vi "Actor Core.vi"(8 "error in":errorcluster, 11 "Panel Actor With Events in":refnum<class "Helper Methods.lvclass">) -> (0 "error out":errorcluster, 3 "Actor out":refnum<class "Actor.lvclass">)   [LabVIEW 2017, in "2. Basic Panel Actors.lvlib" / "Helper Methods.lvclass"]
doc: "The user interface for this panel.\n----\nCopyright: MGI 2016\nAuthor: Derek Trepanier"
uses:
  Helper Methods.lvclass
  <vilib>/ActorFramework/Stop Msg/Stop Msg.lvclass
  panel-manager/Source/MGI-Panel Manager.lvlib
  panel-manager/Source/Panel/Subpanel/Subpanel.vi
  panel-manager/Source/Panel/Subpanel/Subpanel.lvclass
  Description Panel/Description Panel.lvclass
  panel-actors/Source/Panel Actor/Panel Actor.lvclass
  D:/test/LabView_PanelManager/panel-actors/Source/Panel Actor/Panel Actor.lvclass
  D:/test/LabView_PanelManager/panel-manager/Source/Panel/Panel.lvclass
  <vilib>/ActorFramework/Actor/Actor.lvclass
panel:
  out "Initialization Time":string
  out "Latest ID":i32
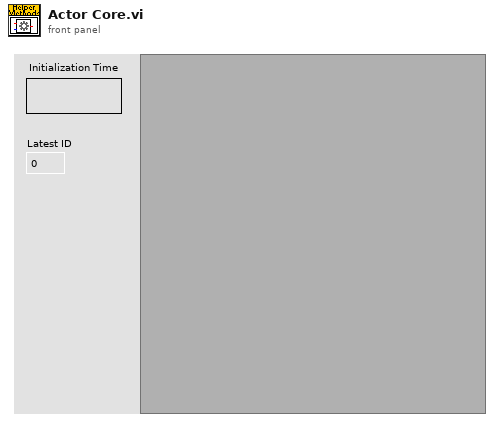
[diagram p1: front panel]
types:
  T1 = cluster{"Event Registration Refnum":refnum<event-registration>, "Pnl Actor":refnum<event-registration>}
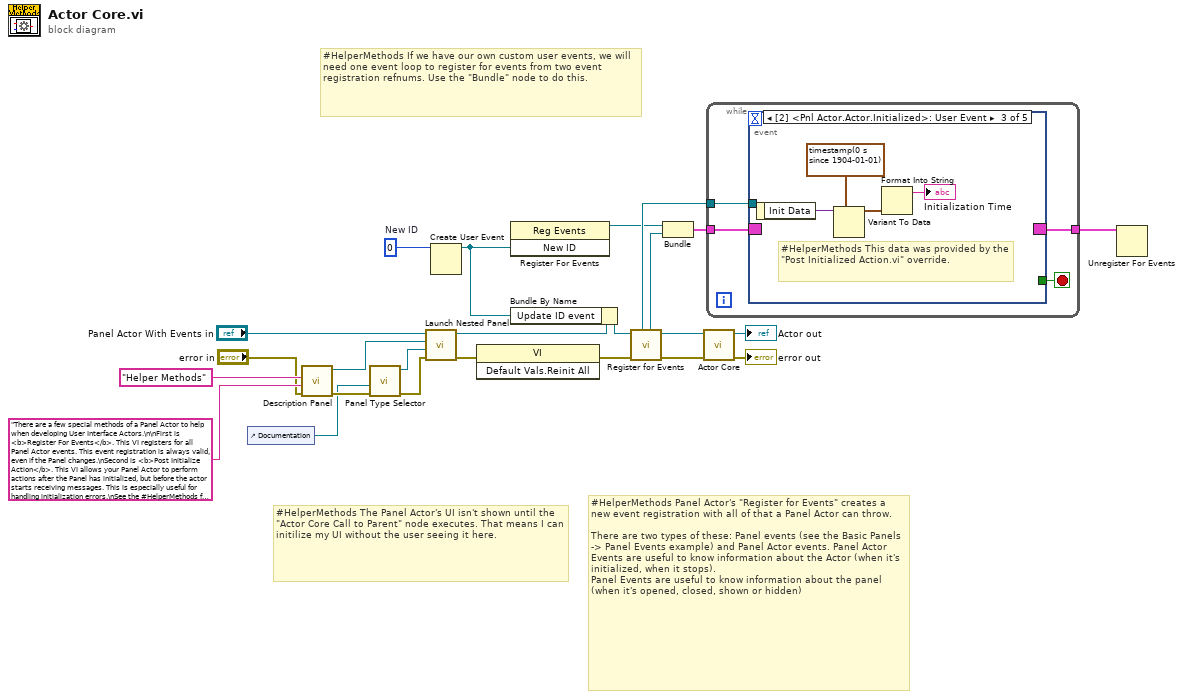
[diagram p0: block diagram]
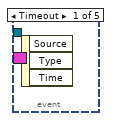
[diagram p2: hidden frame]
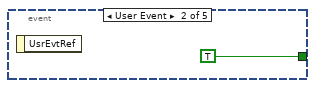
[diagram p3: hidden frame]
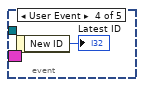
[diagram p4: hidden frame]
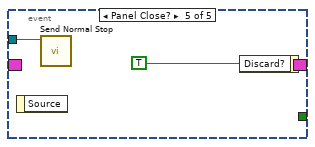
[diagram p5: hidden frame]
diagram:
  w17 = 0  # New ID
  # "#HelperMethods The Panel Actor's UI isn't shown until the \"Actor Core Call to Parent\" node executes. That means I can initilize my UI without the user seeing it here."
  # "#HelperMethods If we have our own custom user events, we will need one event loop to register for events from two event registration refnums. Use the \"Bundle\" node to do this."
  # "#HelperMethods Panel Actor's \"Register for Events\" creates a new event registration with all of that a Panel Actor can throw.\n\nThere are two types of these: Panel events (see the Basic Panels -> Panel Events example) and Panel Actor events. Panel Actor Events are useful to know information about the Actor (when it's initialized, when it stops).\nPanel Events are useful to know information about the panel (when it's opened, closed, shown or hidden)"
  n1 = control-ref of="Documentation"() -> (w1:refnum<vi>)
  n2 = call "Description Panel.vi"("error in (no error)"="error in", "Description"="There are a few special methods of a Panel Actor to help when developing User Interface Actors.\n\nFirst is <b>Register For Events</b>. This VI registers for all Panel Actor events. This event registration is always valid, even if the Panel changes.\nSecond is <b>Post Initialize Action</b>. This VI allows your Panel Actor to perform actions after the Panel has initialized, but before the actor starts receiving messages. This is especially useful for handling initialization errors.\nSee the #HelperMethods for more info.\n" ("Description Title"), "Description Title"="Helper Methods") -> ("error out"=w5:errorcluster, "Description Panel out"=w9:refnum<class "Description Panel.lvclass">)  [unwired: 7 in]
  n3 = call-poly "Panel Type Selector.vi"("Error In"=w5, "Sub Panel"=w1) -> ("Error Out"=w10:errorcluster, "Subpanel Out"=w11:refnum<class "Subpanel.lvclass">)  [unwired: 8 in]
  n4 = call "Launch Nested Panel.vi"("error in (no error)"=w10, "Panel"=w11, "Nested Panel Actor"=w9, "Panel Actor in"="Panel Actor With Events in") -> ("error out"=w2:errorcluster, "Panel Actor out"=w3:refnum<class "Helper Methods.lvclass">)  [unwired: 4 in, 2 out]
  n5 = Create User Event(user event datatype=w17) -> (user event=w13:refnum<user-event>)  [unwired: 1 in, 1 out]
  n6 = invoke class="VI" method="Default Vals.Reinit All"(error in=w2) -> (error out=w12:errorcluster)  [unwired: 2 in, 2 out]
  n7 = register-events(w13) -> (reference out=w15:refnum<event-registration>)  [unwired: 2 in, 1 out]
  n8 = Bundle By Name(cluster=w3, "Update ID event"=w13) -> (w14:refnum<class "Helper Methods.lvclass">)
  n9 = call "Register for Events.vi"("Error In"=w12, "Panel Actor in"=w14) -> ("Error Out"=w20:errorcluster, "Panel Actor out"=w21:refnum<class "Helper Methods.lvclass">, "Pnl Actor"=w19:refnum<event-registration>, "Self Enqueuer"=w18:refnum<class "Message Enqueuer.lvclass">)  [unwired: 5 in, 1 out]
  n10 = Bundle("Event Registration Refnum"=w15, "Pnl Actor"=w19) -> (w16:T1)  [unwired: 1 in]
  n11 = call-parent "Actor Core.vi"("error in"=w20, "Panel Actor in"=w21) -> ("error out"=→"error out":errorcluster, "Actor out"=→"Actor out":refnum<class "Actor.lvclass">)  [unwired: 8 in]
  n12 = while {
    tunnel: w16 -> [w28]
    tunnel: w18 -> [w27]
    tunnel: [w25] -> w22
    stop <- w26 stop-if-true
    n13 = event shown="[2] <Pnl Actor.Actor.Initialized>: User Event" {
      selector: w28 -> [_ _ _ _ _]
      dyn-events: [_ _ _ _ _] -> w25
      timeout: _ -> [_ _ _ _ _]
      tunnel: w27 -> [_ _ _ _ w36]
      tunnel: [_ TRUE _ _ _] -> w26
      event Timeout {
        n14 = event-data() -> ()  [unwired: 1 in, 3 out]
      }
      event User Event {
        n15 = event-data() -> ()  [unwired: 1 in, 1 out]
      }
      event User Event {
        # "#HelperMethods This data was provided by the \"Post Initialized Action.vi\" override."
        n16 = event-data() -> ("Init Data"=w33:variant)  [unwired: 1 in]
        n17 = Variant To Data(type=timestamp(0 s since 1904-01-01), Variant=w33) -> (data=w32:timestamp)  [unwired: 1 in, 1 out]
        n18 = Format Into String(w32) -> (resulting string=→"Initialization Time":string)  [unwired: 3 in, 1 out]
      }
      event User Event {
        n19 = event-data() -> ("New ID"=→"Latest ID":i32)  [unwired: 1 in]
      }
      event Panel Close? {
        n20 = event-data() -> ()  [unwired: 1 in, 1 out]
        n21 = call <vilib>:"Send Normal Stop.vi"("Message Enqueuer"=w36) -> ()  [unwired: 10 in, 1 out]
        n22 = event-data("Discard?"=TRUE) -> ()  [unwired: 1 in, 1 out]
      }
    }
  }
  n23 = Unregister For Events(event registration refnum=w22) -> ()  [unwired: 1 in, 1 out]
